vi "TagContainer-SetLock.vi"(8 "error in (no error)":errorcluster, 10 "Lock?(T)":bool=TRUE, 11 "TagContainer":T1) -> (0 "error out":errorcluster, 3 "TagContainer(dup)":T1)   [LabVIEW 2017, in "TagContainer.lvlib"]
uses:
  TagContainer.lvlib
  Typedef/TagContainer.ctl
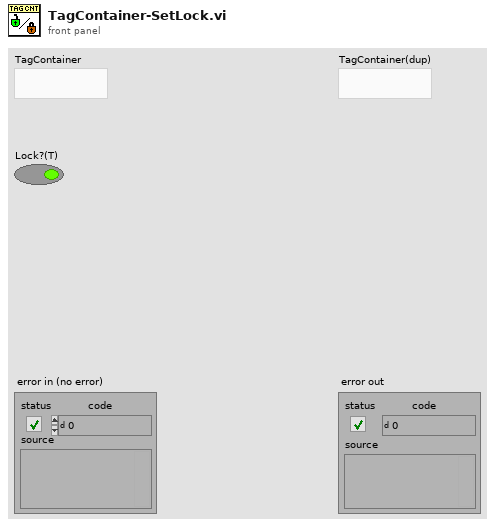
[diagram p1: front panel]
types:
  T1 = typedef "TagContainer.lvlib/TagContainer.ctl" = refnum<k1>
  T2 = typedef "TagContainer.lvlib/tagcontainer-data.ctl" = cluster{"tag-map":variant, "timestamp-map":variant, "namecacher-map":variant, "DataTypeCacher-map":variant, "Tag Adding Lock?":bool, "Global Change Timestamp":timestamp}
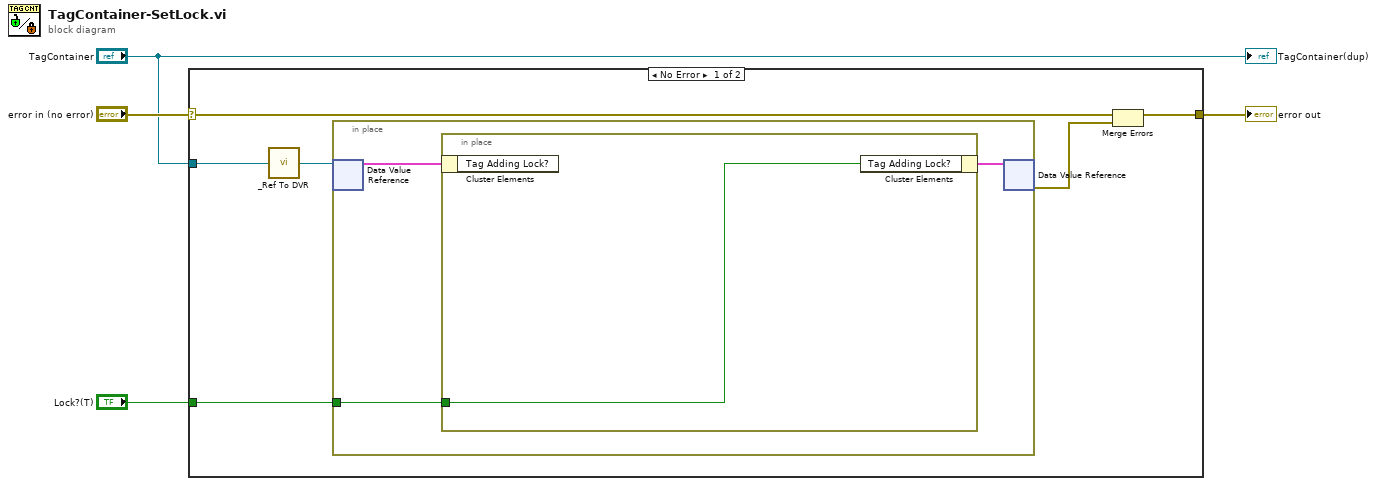
[diagram p0: block diagram]
diagram:
  n1 = case shown="No Error" "error in (no error)" {
    selector: "error in (no error)" -> [w9 w15]
    tunnel: [w10 w15] -> w3
    tunnel: "TagContainer" -> [w7 _]
    tunnel: "Lock?(T)" -> [w5 _]
    frame No Error {
      n2 = call "_Ref To DVR.vi"("TagContainer"=w7) -> ("DVR"=w6:refnum<data-value>)
      n3 = in-place "In Place Element Structure" {
        in-place-border: w5 -> [w13]
        n4 = in-place-dvr #1(w6) -> (w12:T2)  [unwired: 1 out]
        n5 = in-place {
          in-place-border: w13 -> [w14]
          n6 = in-place-cluster #2(w12) -> ()  [unwired: 1 out]
          n7 = in-place-cluster #2("Tag Adding Lock?"=w14) -> (w11:T2)
        }
        n8 = in-place-dvr #1(w11) -> (w8:errorcluster)  [unwired: 1 out]
      }
      n9 = Merge Errors(w9, w8) -> (w10:errorcluster)
    }
    frame Error {
    }
  }
  "error out" <- w3
  "TagContainer(dup)" <- "TagContainer"
